vi "BER.vi"(9 "input reference bit stream":i8[](array[numeric]), 10 "input bit stream":i8[](array[numeric])) -> (2 "ber":dbl)   [LabVIEW 2010]
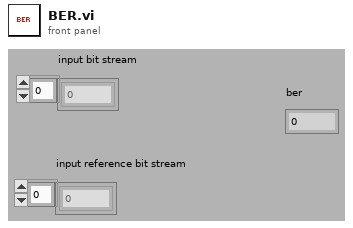
[diagram p1: front panel]
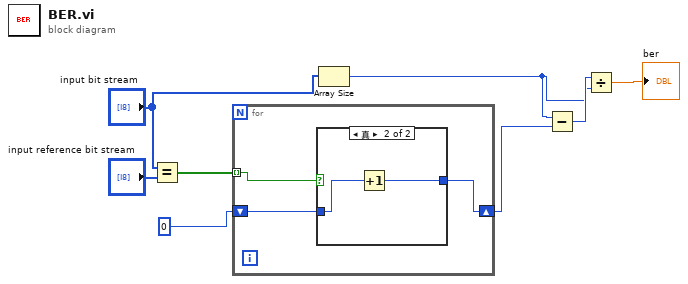
[diagram p0: block diagram]
diagram:
  n1 = Equal?(x="input bit stream", y="input reference bit stream") -> (x = y?=w7:bool[])
  n2 = for {
    tunnel: w7 -> [w10] mode=indexing
    shift-right: [w9] -> w4
    shift-left: 0 -> [w11]
    n3 = case shown="真" w10 {
      tunnel: w11 -> [w12 w14]
      tunnel: [w12 w13] -> w9
      frame False {
      }
      frame True {
        n4 = Increment(x=w14) -> (x+1=w13:i32)
      }
    }
  }
  n5 = Array Size(array="input bit stream") -> (size(s)=w1:i32)
  n6 = Subtract(x=w1, y=w4) -> (x-y=w2:i32)
  n7 = Divide(x=w2, y=w1) -> (x/y=→"ber":dbl)
